vi "Get Frame Type.vi"(8 "error in (no error)":errorcluster caption="entrée d'erreur (pas d'erreur)", 11 "Wait_Frame_ERP1 en entrée":refnum<class "Wait_Frame_ERP1.lvclass">) -> (0 "error out":errorcluster caption="sortie d'erreur", 2 "Frame Type":enum16{"Teach IN", "Normal Mode"}(ring), 3 "Wait_Frame_ERP1 en sortie":refnum<class "Wait_Frame_ERP1.lvclass">)   [LabVIEW 2020, in "Library Test.lvlib" / "Wait_Frame_ERP1.lvclass"]
uses:
  Wait_Frame_ERP1.lvclass
  Wait_Frame_ERP1.lvclass/Wait_Frame_ERP1.ctl
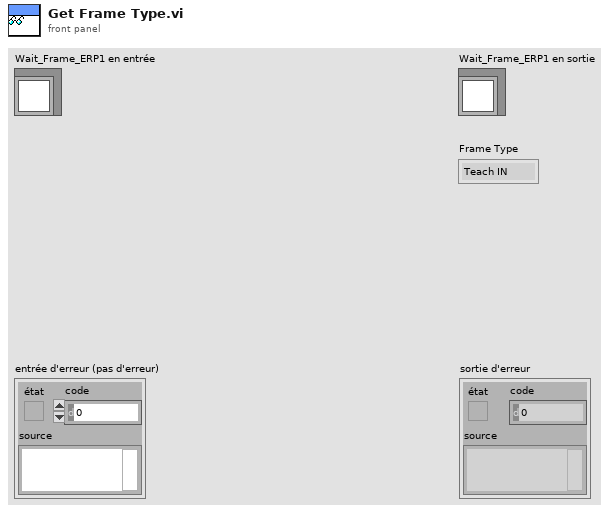
[diagram p1: front panel]
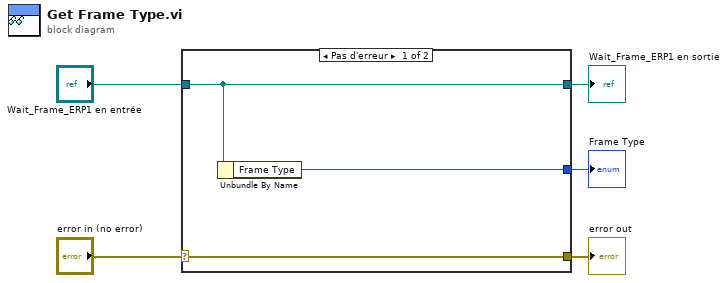
[diagram p0: block diagram]
diagram:
  n1 = case shown="Pas d'erreur" "error in (no error)" {
    selector: "error in (no error)" -> [w8 w9]
    tunnel: [w8 w9] -> w4
    tunnel: [w7 w10] -> w2
    tunnel: "Wait_Frame_ERP1 en entrée" -> [w7 w10]
    tunnel: [w6 _] -> w1
    frame No Error {
      n2 = Unbundle By Name(w7) -> ("Frame Type"=w6:enum16{"Teach IN", "Normal Mode"})
    }
    frame Error {
    }
  }
  "error out" <- w4
  "Wait_Frame_ERP1 en sortie" <- w2
  "Frame Type" <- w1
